vi "FilterScanPar_LS1.vi"(6 "SearchVarPar":bool, 7 "SearchKey":bool, 8 "error in (no error)":errorcluster, 9 "VarParam":string, 10 "ScanParams":T1[](array[typedef]), 11 "KeyWord":string) -> (0 "error out":errorcluster, 3 "ScanParamsOut":T1[](array[typedef]))   [LabVIEW 2012]
uses:
  Interface Class/ScanParams.ctl
  Interface Class/Interface.lvclass
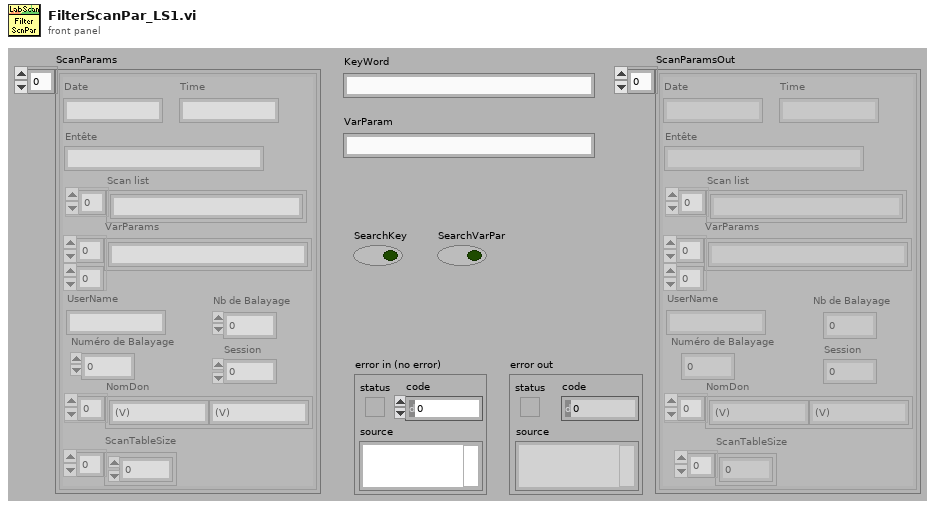
[diagram p1: front panel]
types:
  T1 = typedef "Interface.lvclass/ScanParams.ctl" = cluster{"Entête":string, "Scan list":string[], "NbCourbe":i32, "IndCourbe":i64, "NomDon":string[], "Session ":i32, "Date":string, "Time":string, "VarParams":string[][], "UserName":string, "ScanTableSize":i32[]}
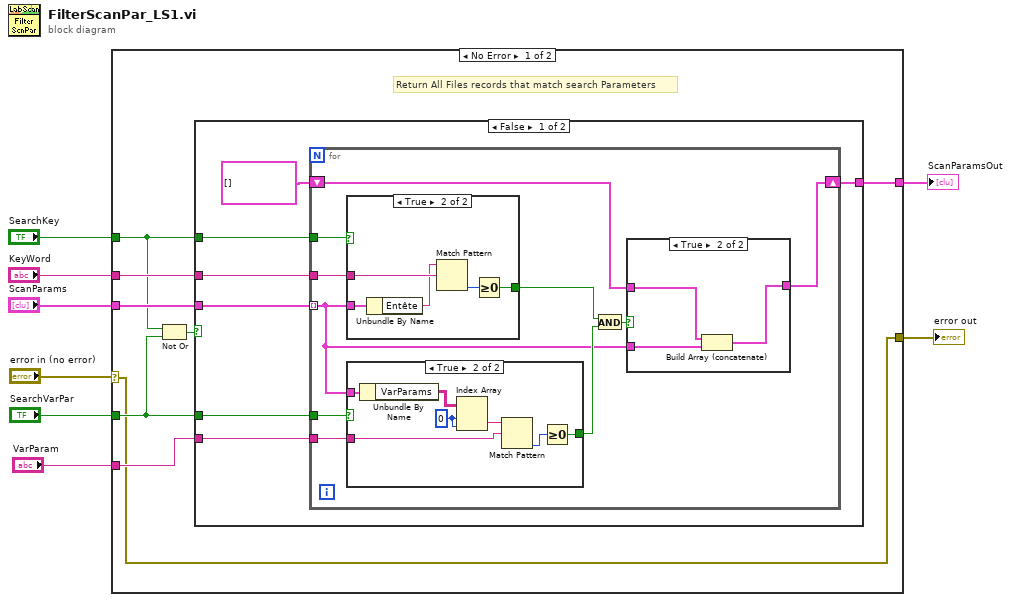
[diagram p0: block diagram]
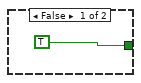
[diagram p3: hidden frame]
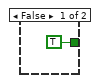
[diagram p4: hidden frame]
diagram:
  n1 = case shown="No Error" "error in (no error)" {
    selector: "error in (no error)" -> [w9 w54]
    tunnel: "KeyWord" -> [w16 _]
    tunnel: "ScanParams" -> [w15 w53]
    tunnel: "SearchKey" -> [w13 _]
    tunnel: "SearchVarPar" -> [w12 _]
    tunnel: [w11 w53] -> w4
    tunnel: "VarParam" -> [w10 _]
    tunnel: [w9 w54] -> w1
    frame No Error {
      # "Return All Files records that match search Parameters"
      n2 = Not Or(1:w12, 2:w13) -> (0:w14:bool)
      n3 = case shown="False" w14 {
        tunnel: w16 -> [w23 _]
        tunnel: w15 -> [w22 w52]
        tunnel: w13 -> [w20 _]
        tunnel: w12 -> [w19 _]
        tunnel: [w17 w52] -> w11
        tunnel: w10 -> [w18 _]
        frame False {
          n4 = for {
            tunnel: w22 -> [w25] mode=indexing
            tunnel: w23 -> [w33]
            shift-right: [w24] -> w17
            shift-left: T1[] [] -> [w29]
            tunnel: w20 -> [w31]
            tunnel: w19 -> [w32]
            tunnel: w18 -> [w30]
            n5 = case shown="True" w31 {
              tunnel: w33 -> [_ w51]
              tunnel: w25 -> [_ w48]
              tunnel: [TRUE w47] -> w28
              frame False {
              }
              frame True {
                n6 = Unbundle By Name(w48) -> ("Entête"=w50:string)
                n7 = Match Pattern(string=w50, regular expression=w51) -> (offset past match=w49:i32)  [unwired: 1 in, 3 out]
                n8 = Greater Or Equal To 0?(x=w49) -> (x >= 0?=w47:bool)
              }
            }
            n9 = case shown="True" w32 {
              tunnel: w25 -> [_ w45]
              tunnel: w30 -> [_ w41]
              tunnel: [TRUE w40] -> w27
              frame False {
              }
              frame True {
                w43 = 0 ("indice (ligne)")
                n10 = Unbundle By Name(w45) -> ("VarParams"=w44:string[][])
                n11 = Index Array(array=w44, index (row)=w43, index (col)=w43) -> (element=w42:string)
                n12 = Match Pattern(string=w42, regular expression=w41) -> (offset past match=w39:i32)  [unwired: 1 in, 3 out]
                n13 = Greater Or Equal To 0?(x=w39) -> (x >= 0?=w40:bool)
              }
            }
            n14 = And(x=w28, y=w27) -> (x .and. y?=w26:bool)
            n15 = case shown="True" w26 {
              tunnel: [w34 w37] -> w24
              tunnel: w29 -> [w34 w35]
              tunnel: w25 -> [_ w36]
              frame False {
              }
              frame True {
                n16 = Build Array (concatenate)(w35, w36) -> (w37:T1[])
              }
            }
          }
        }
        frame True {
          # "No search parameter supplied"
        }
      }
    }
    frame Error {
    }
  }
  "error out" <- w1
  "ScanParamsOut" <- w4
